vi "DO Reset LV2G.vi"(0 "Task":enum16{"Init", "Write", "Read"}(ring)=enum."Read", 5 "Write":bool, 7 "DO Data":bool[](array[boolean]), 9 "DO Data 1":bool[](array[boolean]), 11 "error in":errorcluster) -> (4 "Read":bool, 6 "DO Data":bool[](array[boolean]), 8 "DO Data 1":bool[](array[boolean]), 15 "error out":errorcluster)   [LabVIEW 2023, in "GUI.lvlib" / "Diagnostic.lvlib" / "Diagnostic.lvclass"]
uses:
  Diagnostic.lvclass
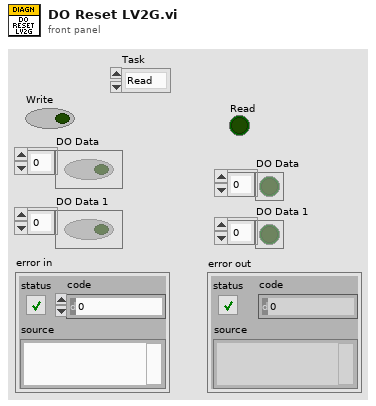
[diagram p1: front panel]
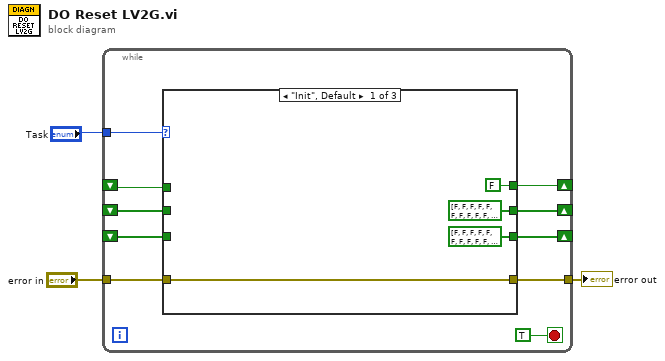
[diagram p0: block diagram]
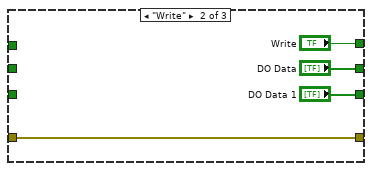
[diagram p2: hidden frame]
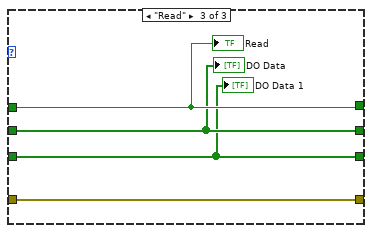
[diagram p3: hidden frame]
diagram:
  n1 = while {
    tunnel: "Task" -> [w12]
    shift-right: [w11] -> _
    shift-left: _ -> [w10]
    tunnel: "error in" -> [w9]
    tunnel: [w8] -> w1
    shift-right: [w6] -> _
    shift-left: _ -> [w4]
    shift-right: [w7] -> _
    shift-left: _ -> [w5]
    stop <- TRUE stop-if-true
    n2 = case shown="\"Init\", Default" w12 {
      tunnel: [FALSE "Write" w25] -> w11
      tunnel: w10 -> [_ _ w25]
      tunnel: w9 -> [w16 w20 w24]
      tunnel: [w16 w20 w24] -> w8
      tunnel: [bool[] [FALSE, FALSE, FALSE, FALSE, FALSE, FALSE, FALSE, FALSE, FALSE, FALSE, FALSE, FALSE, FALSE, FALSE, FALSE, FALSE, FALSE, FALSE, FALSE, FALSE, FALSE, FALSE, FALSE, FALSE, FALSE, FALSE, FALSE, FALSE, FALSE, FALSE, FALSE, FALSE] ("DO Data") "DO Data" w23] -> w7
      tunnel: [bool[] [FALSE, FALSE, FALSE, FALSE, FALSE, FALSE, FALSE, FALSE, FALSE, FALSE, FALSE, FALSE, FALSE, FALSE, FALSE, FALSE, FALSE, FALSE, FALSE, FALSE, FALSE, FALSE, FALSE, FALSE, FALSE, FALSE, FALSE, FALSE, FALSE, FALSE, FALSE, FALSE, FALSE, FALSE, FALSE, FALSE, FALSE, FALSE, FALSE, FALSE] ("DO Data 1") "DO Data 1" w22] -> w6
      tunnel: w5 -> [_ _ w23]
      tunnel: w4 -> [_ _ w22]
      frame "Init", Default {
      }
      frame "Write" {
      }
      frame "Read" {
        "Read" <- w25
        "DO Data" <- w23
        "DO Data 1" <- w22
      }
    }
  }
  "error out" <- w1
